vi "Set Scaling Parameters (Polynomial).vi"(0 "session in":refnum<k21>, 1 "serial number":string, 2 "password":string, 5 "physical channel":refnum<k21>="$DefaultPhysChans", 7 "forward coefficients":dbl[](array[numeric]), 9 "reverse coefficients":dbl[](array[numeric]), 11 "error in (no error)":errorcluster) -> (4 "session out":refnum<k21>, 6 "physical channel out":refnum<k21>, 15 "error out":errorcluster)   [LabVIEW 2020, in "SLSC.lvlib"]
doc: "Sets scaling parameters for a polynomial scale that uses an nth order polynomial equation. A polynomial scale contains both a polynomial to convert pre-scaled values to scaled values and a polynomial to convert scaled values to pre-scaled values."
uses:
  <vilib>/SLSC/SLSC.lvlib
  nislsclvapi.dll
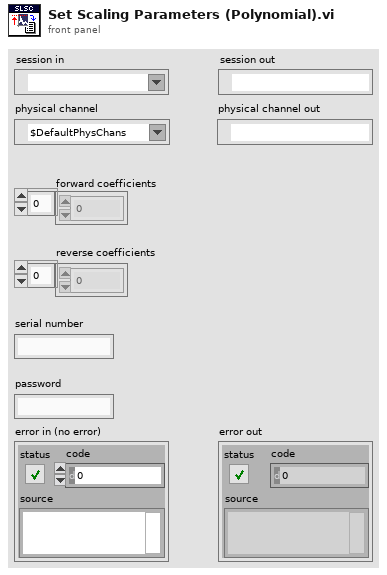
[diagram p1: front panel]
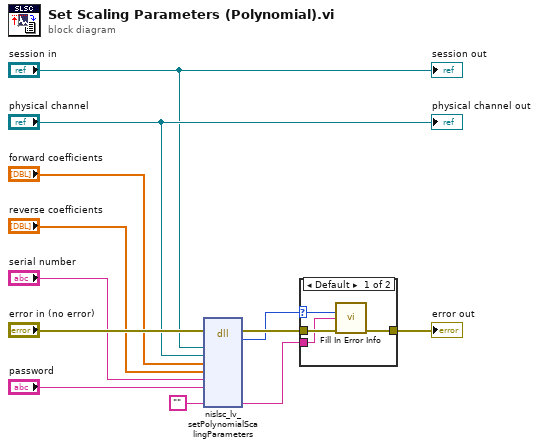
[diagram p0: block diagram]
diagram:
  n1 = dll-call lib="nislsclvapi.*" fn="nislsc_lv_setPolynomialScalingParameters"(error in="error in (no error)", "session"="session in", "physical channel"="physical channel", "forwardCoeffs"="forward coefficients", "reverseCoeffs"="reverse coefficients", "serialNum"="serial number", "password"="password", "extendedErrorInfo"="") -> (error out=w4:errorcluster, "return type"=w2:i32, "extendedErrorInfo"=w3:string)  [unwired: 10 in, 1 out]
  n2 = case shown="Default" w2 {
    selector: w2 -> [w13 _]
    tunnel: w3 -> [w14 _]
    tunnel: w4 -> [w16 w17]
    tunnel: [w15 w17] -> w1
    frame Default {
      n3 = call <vilib>:"Fill In Error Info.vi"("status code"=w13, "extended error info"=w14, "error in"=w16) -> ("error out"=w15:errorcluster)  [unwired: 12 in]
    }
    frame 0 {
    }
  }
  "error out" <- w1
  "session out" <- "session in"
  "physical channel out" <- "physical channel"
